vi "F8588A Configure Sampling.vi"(0 "VISA resource in":refnum<visa-resource-name>, 1 "sample period [s] (-1: use EXT trig as source)":dbl=-1.0 format="%#_6p", 2 "apperture [s] (1.4us)":dbl=1.4e-06 format="%#_6p", 3 "LEVEL trigger":T1 caption="Cluster", 4 "EXT OUT signal (APER)":T2, 5 "error in":errorcluster, 6 "range [V] (10V)":dbl=10.0, 7 "samples count (100)":i32=100, 11 "delay [s]":dbl=1e-07, 12 "stream mode (False)":bool, 13 "first sample (AUTO)":T3) -> (14 "VISA resource name out":refnum<visa-resource-name>, 19 "error out":errorcluster)   [LabVIEW 2013]
doc: "This VI configures DMM for digitizing of sequence of samples. It will enable the mode (DCV, DSDC, DSAC), then it will decide sample clocking source (TIMER or EXT), decides format of memory/data transfer based on aperture (SINT, DINT) and puts the meter in TARM HOLD mode so it is ready to start when DMM is armed. When stream mode is enabled it disables memory so the data will be sent directly to the controller. Frist sample input specifies what is used as trigger source. Default is AUTO. For stream mode SYN mode is convenient because it will trigger when controller is ready to receive.\n\nNote: Reentrant VI so it can be executed in parallel for multiple 3458A sessions."
uses:
  DMM/3458A Digitizing Low Levels/Configure/First Sample Trigger.ctl
  DMM/3458A Digitizing Low Levels/Configure/EXT OUT mode.ctl
  DMM/3458A Digitizing Low Levels/Configure/Level Setup.ctl
  DMM/3458A Digitizing Low Levels/3458A Digitizing Low Levels.lvlib
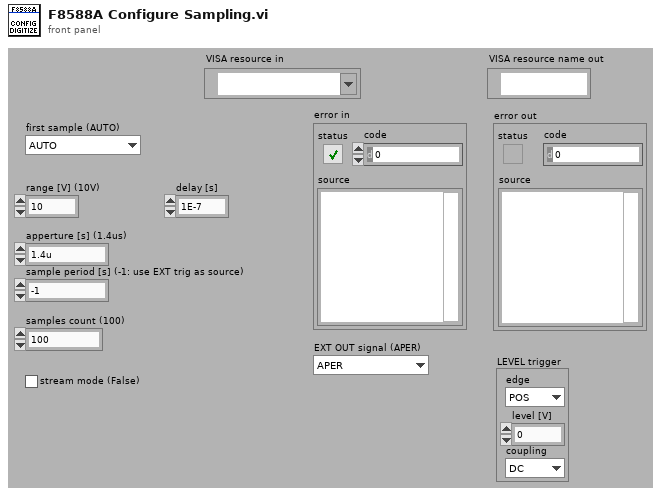
[diagram p1: front panel]
types:
  T1 = typedef "3458A Virtual Digitizer.lvlib/3458A Digitizing Low Levels.lvlib/Level Setup.ctl" = cluster{"edge":enum16{"POS", "NEG"}, "level [V]":dbl, "coupling":enum16{"DC", "AC"}}
  T2 = typedef "3458A Virtual Digitizer.lvlib/3458A Digitizing Low Levels.lvlib/EXT OUT mode.ctl" = enum16{"APER", "ICOMP"}
  T3 = typedef "3458A Virtual Digitizer.lvlib/3458A Digitizing Low Levels.lvlib/First Sample Trigger.ctl" = enum16{"AUTO", "EXT", "SYN", "SGL", "HOLD", "LEVEL"}
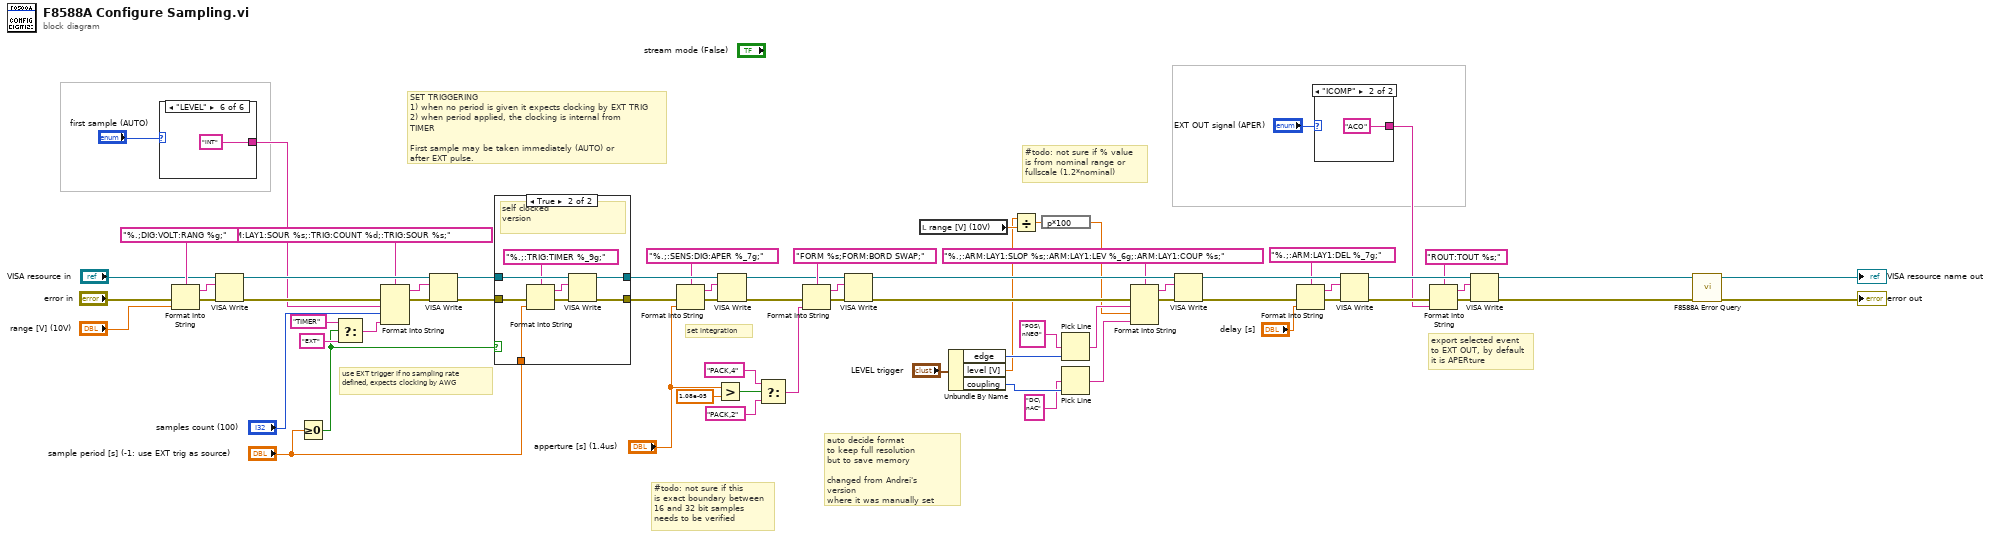
[diagram p0: block diagram]
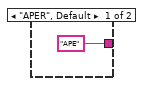
[diagram p2: hidden frame]
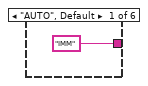
[diagram p3: hidden frame]
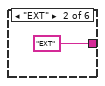
[diagram p4: hidden frame]
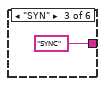
[diagram p5: hidden frame]
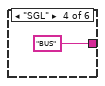
[diagram p6: hidden frame]
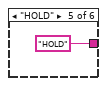
[diagram p7: hidden frame]
diagram:
  # "#todo: not sure if % value\nis from nominal range or \nfullscale (1.2*nominal)"
  # "export selected event\nto EXT OUT, by default\nit is APERture"
  # "#todo: not sure if this\nis exact boundary between\n16 and 32 bit samples\nneeds to be verified"
  # "auto decide format\nto keep full resolution\nbut to save memory\n\nchanged from Andrei's version\nwhere it was manually set"
  # "set integration"
  # "use EXT trigger if no sampling rate\ndefined, expects clocking by AWG"
  # "SET TRIGGERING\n1) when no period is given it expects clocking by EXT TRIG\n2) when period applied, the clocking is internal from TIMER\n\nFirst sample may be taken immediately (AUTO) or \nafter EXT pulse."
  n1 = case shown="\"LEVEL\"" "first sample (AUTO)" {
    tunnel: ["IMM" "EXT" "SYNC" "BUS" "HOLD" "INT"] -> w6
    frame "AUTO", Default {
    }
    frame "EXT" {
    }
    frame "SYN" {
    }
    frame "SGL" {
    }
    frame "HOLD" {
    }
    frame "LEVEL" {
    }
  }
  n2 = Format Into String(format string="%.;DIG:VOLT:RANG %g;" ("write buffer"), error in="error in", "range [V] (10V)") -> (resulting string=w69:string, error out=w70:errorcluster)  [unwired: 1 in]
  n3 = VISA Write(VISA resource name="VISA resource in", write buffer=w69, error in (no error)=w70) -> (VISA resource name out=w67:refnum<visa-resource-name>, error out=w59:errorcluster)  [unwired: 1 out]
  n4 = Greater Or Equal To 0?(x="sample period [s] (-1: use EXT trig as source)") -> (x >= 0?=w55:bool)
  n5 = Select(t="TIMER" ("multi-line string"), s=w55, f="EXT" ("multi-line string")) -> (s? t:f=w60:string)
  n6 = Format Into String(format string=":ARM:LAY2:SOUR IMM;:ARM:LAY1:SOUR %s;:TRIG:COUNT %d;:TRIG:SOUR %s;", error in=w59, w6, "samples count (100)", w60) -> (resulting string=w64:string, error out=w66:errorcluster)  [unwired: 1 in]
  n7 = VISA Write(VISA resource name=w67, write buffer=w64, error in (no error)=w66) -> (VISA resource name out=w57:refnum<visa-resource-name>, error out=w58:errorcluster)  [unwired: 1 out]
  n8 = case shown="True" w55 {
    tunnel: w58 -> [w77 w86]
    tunnel: w57 -> [w78 w84]
    tunnel: "sample period [s] (-1: use EXT trig as source)" -> [_ w82]
    tunnel: [w77 w81] -> w52
    tunnel: [w78 w80] -> w51
    frame False {
      # "EXT clocked"
    }
    frame True {
      # "self clocked\nversion"
      n9 = Format Into String(format string="%.;:TRIG:TIMER %_9g;" ("write buffer"), error in=w86, w82) -> (resulting string=w79:string, error out=w85:errorcluster)  [unwired: 1 in]
      n10 = VISA Write(VISA resource name=w84, write buffer=w79, error in (no error)=w85) -> (VISA resource name out=w80:refnum<visa-resource-name>, error out=w81:errorcluster)  [unwired: 1 out]
    }
  }
  n11 = Format Into String(format string="%.;:SENS:DIG:APER %_7g;", error in=w52, "apperture [s] (1.4us)") -> (resulting string=w54:string, error out=w53:errorcluster)  [unwired: 1 in]
  n12 = Greater?(x="apperture [s] (1.4us)", y=1.08e-05) -> (0:w42:bool)
  n13 = VISA Write(VISA resource name=w51, write buffer=w54, error in (no error)=w53) -> (VISA resource name out=w47:refnum<visa-resource-name>, error out=w46:errorcluster)  [unwired: 1 out]
  n14 = Select(t="PACK,4" ("format string"), s=w42, f="PACK,2" ("format string")) -> (s? t:f=w1:string)
  n15 = Format Into String(format string="FORM %s;FORM:BORD SWAP;" ("write buffer"), error in=w46, w1) -> (resulting string=w49:string, error out=w50:errorcluster)  [unwired: 1 in]
  n16 = VISA Write(VISA resource name=w47, write buffer=w49, error in (no error)=w50) -> (VISA resource name out=w25:refnum<visa-resource-name>, error out=w22:errorcluster)  [unwired: 1 out]
  n17 = local read "range [V] (10V)"() -> (w13:dbl)
  n18 = Unbundle By Name("LEVEL trigger") -> ("edge"=w19:enum16{"POS", "NEG"}, "level [V]"=w12:dbl, "coupling"=w17:enum16{"DC", "AC"})
  n19 = Divide(x=w12, y=w13) -> (x/y=w11:dbl)
  n20 = expression code="p*100"(w11) -> (w10:dbl)
  n21 = Pick Line(multi-line string="POS\nNEG" ("string (\"\")"), line index=w19) -> (output string=w18:string)  [unwired: 1 in]
  n22 = Pick Line(multi-line string="DC\nAC" ("string (\"\")"), line index=w17) -> (output string=w16:string)  [unwired: 1 in]
  n23 = Format Into String(format string="%.;:ARM:LAY1:SLOP %s;:ARM:LAY1:LEV %_6g;:ARM:LAY1:COUP %s;" ("write buffer"), error in=w22, w18, w10, w16) -> (resulting string=w21:string, error out=w23:errorcluster)  [unwired: 1 in]
  n24 = VISA Write(VISA resource name=w25, write buffer=w21, error in (no error)=w23) -> (VISA resource name out=w36:refnum<visa-resource-name>, error out=w33:errorcluster)  [unwired: 1 out]
  n25 = Format Into String(format string="%.;:ARM:LAY1:DEL %_7g;" ("write buffer"), error in=w33, "delay [s]") -> (resulting string=w34:string, error out=w35:errorcluster)  [unwired: 1 in]
  n26 = case shown="\"ICOMP\"" "EXT OUT signal (APER)" {
    tunnel: ["APE" "ACO"] -> w2
    frame "APER", Default {
    }
    frame "ICOMP" {
    }
  }
  n27 = VISA Write(VISA resource name=w36, write buffer=w34, error in (no error)=w35) -> (VISA resource name out=w28:refnum<visa-resource-name>, error out=w30:errorcluster)  [unwired: 1 out]
  n28 = Format Into String(format string="ROUT:TOUT %s;" ("write buffer"), error in=w30, w2) -> (resulting string=w27:string, error out=w29:errorcluster)  [unwired: 1 in]
  n29 = VISA Write(VISA resource name=w28, write buffer=w27, error in (no error)=w29) -> (VISA resource name out=w4:refnum<visa-resource-name>, error out=w5:errorcluster)  [unwired: 1 out]
  n30 = call "F8588A Error Query.vi"("error in (no error)"=w5, "VISA resource name"=w4) -> ("error out"=→"error out":errorcluster, "VISA resource name out"=→"VISA resource name out":refnum<visa-resource-name>)  [unwired: 6 in, 2 out]
